vi "IGC100 Advanced Settings.vi"() -> ()   [LabVIEW 2018]
uses:
  <vilib>/Utility/file.llb/Write To Spreadsheet File (string).vi
panel:
  in  "Config File":path=path "C:/Users/Admin/Documents/IPES Control Panel/IPES Config Files/Pressure Log.conf"
  in  "Stop":bool caption="(Safe Stop)"
  in  "Set Defaults":bool
  in  "File Extension":string=".press"
  in  "Filename":string="%Y-%m-%d"
  in  "Path":path=path "C:/Users/dhawthor/Desktop/Pressure Logs"
  # "To permanently change the config file location, first open this VI in a separate instance.  Then stop the VI using Abort (stop sign button) and use \"Right Click\" >> \"Data Operations\" >> \"Make Current Value Default.\""
  # "These control the default values used when saving pressure logs.  To change them, click \"Save Changes\" and they will be updated in the config file."
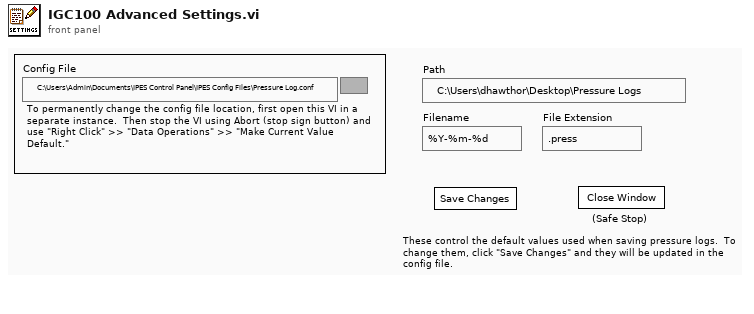
[diagram p1: front panel]
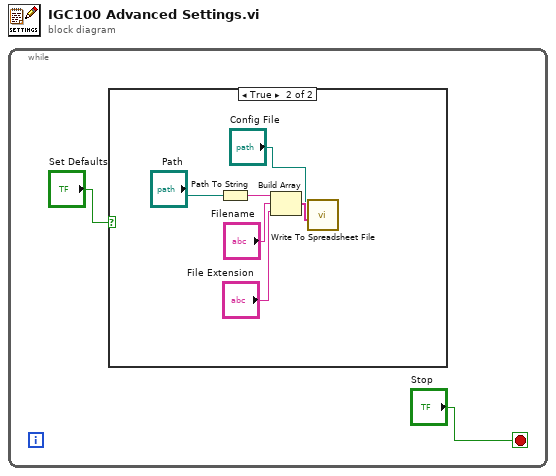
[diagram p0: block diagram]
diagram:
  n1 = while {
    stop <- "Stop" stop-if-true
    n2 = case shown="True" "Set Defaults" {
      frame False {
      }
      frame True {
        n3 = Path To String(path="Path") -> (string=w4:string)
        n4 = Build Array(w4, "Filename", "File Extension") -> (w6:string[])
        n5 = call-poly <vilib>:"Write To Spreadsheet File.vi"("1D data"=w6, "file path (dialog if empty)"="Config File") -> ()  [unwired: 6 in, 1 out]
      }
    }
  }
